vi "Initialize.vi"(0 "Tektronix PA1000 in":refnum<class "Tektronix PA1000.lvclass">, 7 "Reset (T: Reset)":bool=TRUE, 9 "ID Query (T: Check)":bool=TRUE, 11 "error in (no error)":errorcluster) -> (4 "Tektronix PA1000 out":refnum<class "Tektronix PA1000.lvclass">, 6 "VISA resource name":refnum<visa-resource-name>, 15 "error out":errorcluster)   [LabVIEW 2013, in "Universal Power Meter.lvlib" / "Tektronix PA1000.lvlib" / "Tektronix PA1000.lvclass"]
uses:
  Tektronix PA1000.lvclass
  Universal Power Meter class/Universal Power Meter.lvclass
  <instrlib>/Tektronix PA1000/Tektronix PA1000.lvlib
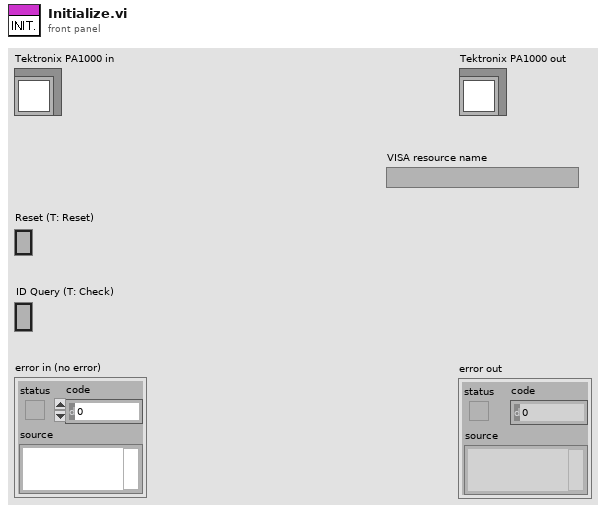
[diagram p1: front panel]
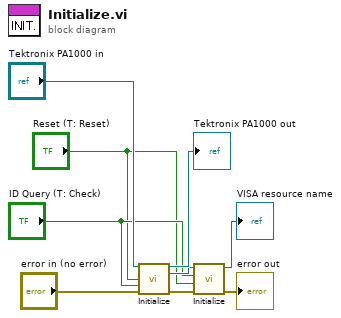
[diagram p0: block diagram]
diagram:
  n1 = call-parent <instrlib>:"Initialize.vi"("Universal Power Meter in"="Tektronix PA1000 in", "Reset (T: Reset)"="Reset (T: Reset)", "ID Query (T: Check)"="ID Query (T: Check)", "error in (no error)"="error in (no error)") -> ("Universal Power Meter out"=→"Tektronix PA1000 out":refnum<class "Tektronix PA1000.lvclass">, "VISA resource name"=w4:refnum<visa-resource-name>, "error out"=w3:errorcluster)  [unwired: 9 in]
  n2 = call <instrlib>:"Initialize.vi"("error in (no error)"=w3, "Reset (True)"="Reset (T: Reset)", "ID Query (True)"="ID Query (T: Check)", "VISA resource name"=w4) -> ("error out"=→"error out":errorcluster, "VISA resource name out"=→"VISA resource name":refnum<visa-resource-name>)  [unwired: 6 in]
